vi "ManStatusPressureGauge.vi"(7 "DriverSettings in":T4, 8 "Error In":errorcluster, 11 "Manometr in":T5 {"MANOMETR" scale=0.0..10.0 scale format="%.1f"}) -> (0 "Error Out":errorcluster, 5 "DriverSettings out":T4)   [LabVIEW 2018]
uses:
  PressureGauge.ctl
  MOKO_LabViewLibrary/MokoLowLevel/MokoLowLovelControl/MLLC_InterfaceType.ctl
  MOKO_LabViewLibrary/MokoLowLevel/MokoLowLovelControl/MLLC_InterfaceSettings.ctl
  MOKO_LabViewLibrary/MokoLowLevel/MokoLowLovelControl/MLLC_InterfaceKind.ctl
panel:
  in  "Cancel Button":bool
  out "message out":string caption="String"
  out "Manometr out":T5 {"MANOMETR" scale=0.0..10.0 scale format="%.1f"}
  in  "завершить":bool
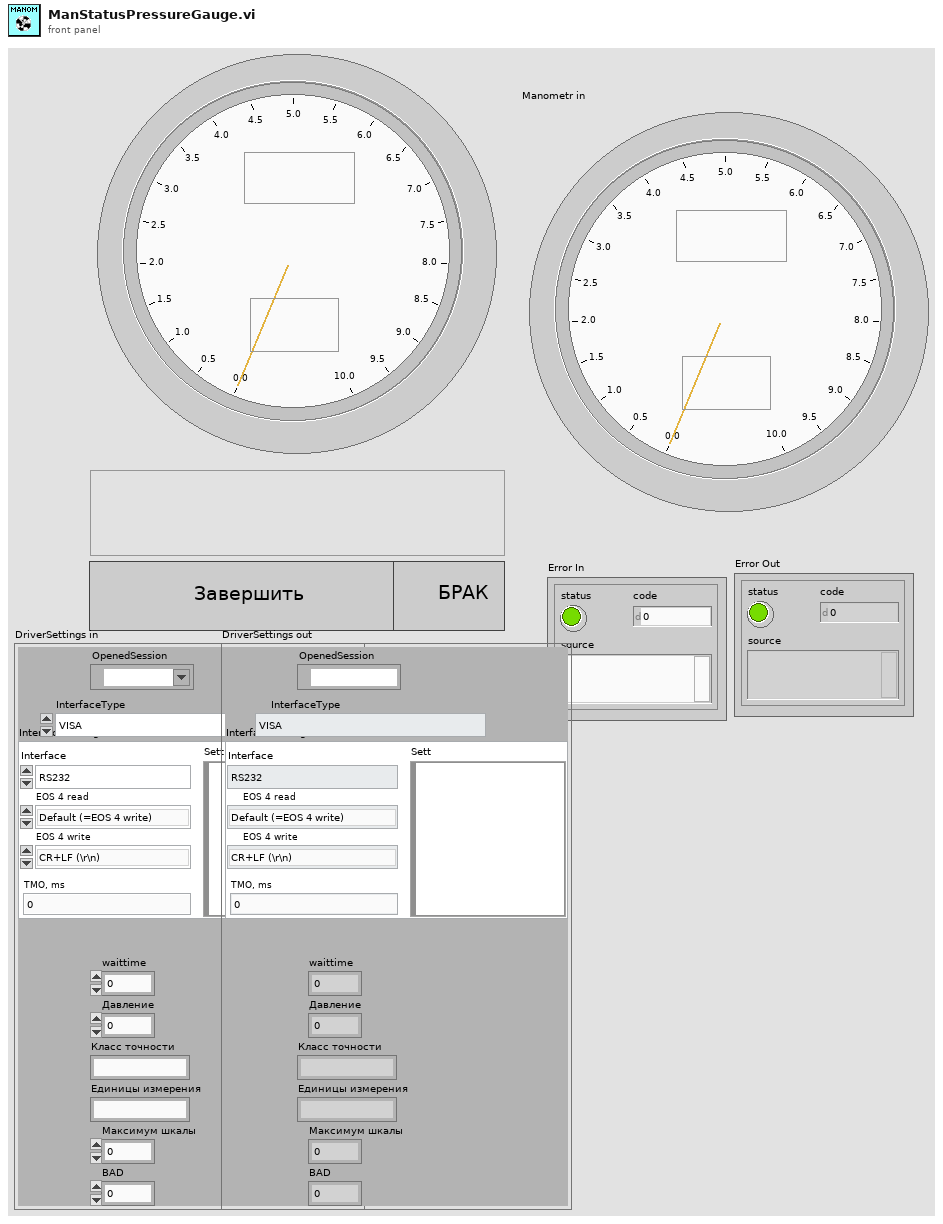
[diagram p1: front panel]
types:
  T1 = typedef "MLLC_InterfaceType.ctl" = enum16{"VISA", "Prologix USB-GPIB"}
  T2 = typedef "MLLC_InterfaceSettings.ctl" = cluster{"Interface":T3, "EOS 4 read":enum16{"Default (=EOS 4 write)", "CR (\\r)", "LF (\\n)", "None"}, "EOS 4 write":enum16{"CR+LF (\\r\\n)", "CR (\\r)", "LF (\\n)", "None"}, "TMO, ms":i32, "Sett":variant}
  T3 = typedef "MLLC_InterfaceKind.ctl" = enum16{"RS232", "GPIB", "USB", "Ethernet", "another"}
  T4 = cluster{"OpenedSession":refnum<visa-resource-name>, "InterfaceType":T1, "InterfaceSettings":T2, "waittime":dbl, "Давление":dbl, "Класс точности":string, "Единицы измерения":string, "Максимум шкалы":dbl, "BAD":dbl}
  T5 = typedef "PressureGauge.ctl" = cluster{"MANOMETR":dbl, "Единица измерения":string, "Класс точности":string, "Максимум шкалы":dbl}
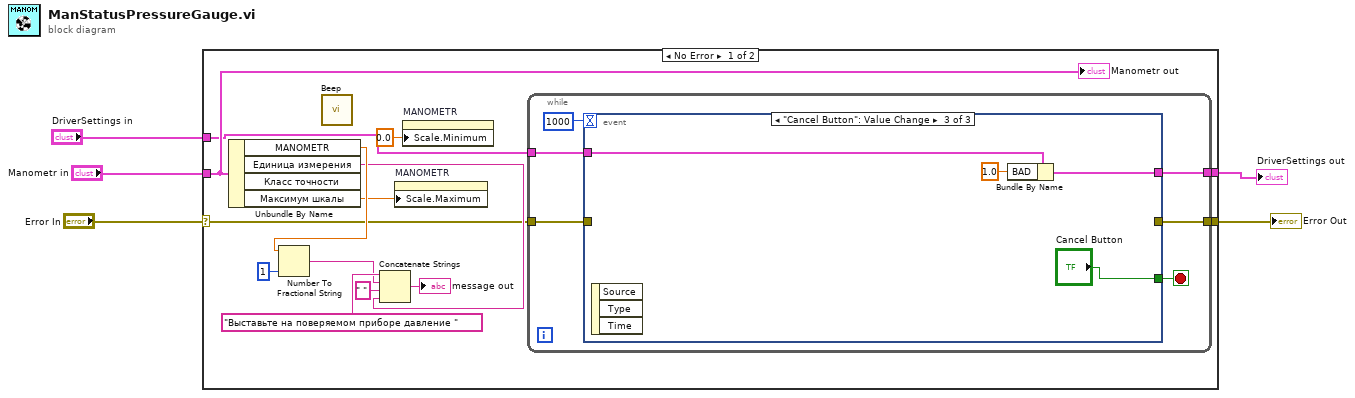
[diagram p0: block diagram]
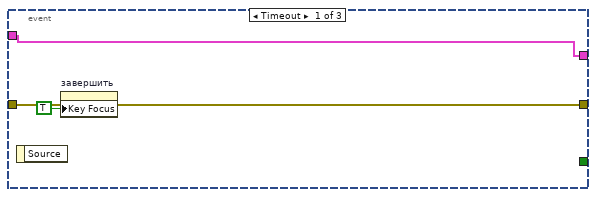
[diagram p2: hidden frame]
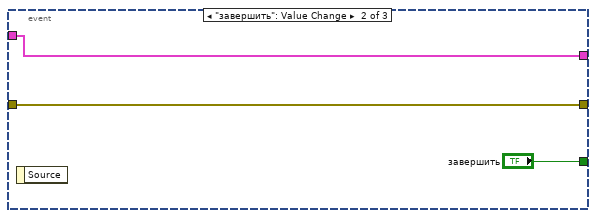
[diagram p3: hidden frame]
diagram:
  n1 = case shown="No Error" "Error In" {
    selector: "Error In" -> [w12 w37]
    tunnel: "Manometr in" -> [w19 _]
    tunnel: [w13 w37] -> w3
    tunnel: [w7 w36] -> w2
    tunnel: "DriverSettings in" -> [w6 w36]
    frame No Error {
      n2 = Unbundle By Name(w19) -> ("MANOMETR"=w18:dbl, "Единица измерения"=w16:string, "Максимум шкалы"=w9:dbl)  [unwired: 1 out]
      n3 = Number To Fractional String(number=w18, precision (6)=i16 1) -> (F-format string=w10:string)  [unwired: 2 in]
      n4 = call <vilib>:"Beep.vi"() -> ()  [unwired: 12 in]
      n5 = Concatenate Strings("Выставьте на поверяемом приборе давление " ("message in"), w10, " " ("string"), w16) -> (→"message out":string)
      n6 = property on="MANOMETR" class="Knob (strict)"("Scale.Maximum"=w9) -> ()  [unwired: 2 in, 2 out]
      n7 = property on="MANOMETR" class="Knob (strict)"("Scale.Minimum"=0.0 ("Scale.Range:Minimum")) -> ()  [unwired: 2 in, 2 out]
      n8 = while {
        tunnel: [w23] -> w13
        tunnel: w12 -> [w22]
        tunnel: [w21] -> w7
        tunnel: w6 -> [w20]
        stop <- w24 stop-if-true
        n9 = event shown="[2] \"Cancel Button\": Value Change" {
          selector: _ -> [_ _ _]
          dyn-events: _ -> [_ _ _]
          timeout: 1000 -> [_ _ _]
          tunnel: [_ "завершить" "Cancel Button"] -> w24
          tunnel: [w27 w30 _] -> w23
          tunnel: w22 -> [w27 w30 _]
          tunnel: [w26 w29 w33] -> w21
          tunnel: w20 -> [w26 w29 w34]
          event Timeout {
            n10 = event-data() -> ()  [unwired: 1 in, 1 out]
            n11 = property on="завершить" class="Bool"("Key Focus"=TRUE) -> ()  [unwired: 2 in, 2 out]
          }
          event "завершить": Value Change {
            n12 = event-data() -> ()  [unwired: 1 in, 1 out]
          }
          event "Cancel Button": Value Change {
            n13 = event-data() -> ()  [unwired: 1 in, 3 out]
            n14 = Bundle By Name(cluster=w34, "BAD"=1.0) -> (w33:T4)
          }
        }
      }
      "Manometr out" <- w19
    }
    frame Error {
    }
  }
  "Error Out" <- w3
  "DriverSettings out" <- w2
